vi "Write.vi"(8 "error in (no error)":errorcluster, 10 "Statement":T1={"timestamp"=timestamp(0 s since 1904-01-01), "level"=enum."INFO", "sourceTag"="", "originVI"="", "message"=""}, 11 "RelayAppender in":refnum<class "RelayAppender.lvclass">) -> (0 "error out":errorcluster, 3 "RelayAppender out":refnum<class "RelayAppender.lvclass">)   [LabVIEW 2026, in "Lumberjack.lvlib" / "RelayAppender.lvclass"]
doc: "Deliver one accepted Statement to the sink. Called by HandleStatement after the statement passes the appender threshold and filter. Receives the structured Statement (not a formatted string): text sinks format via their own Layout here; the relay forwards or enqueues the Statement object. Abstract. DD, must override."
uses:
  RelayAppender.lvclass
  TypeDefs/Statement.ctl
  TypeDefs/Severity.ctl
  RelayAppender.lvclass/RelayAppender.ctl
  Messages/LogStatementMsg.lvclass/LogStatementMsg.lvclass
  Lumberjack.lvlib
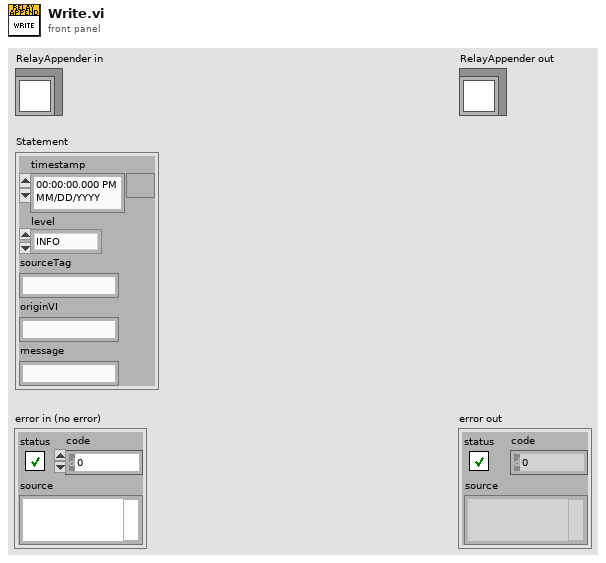
[diagram p1: front panel]
types:
  T1 = typedef "Lumberjack.lvlib/Statement.ctl" = cluster{"timestamp":timestamp, "level":T2, "sourceTag":string, "originVI":string, "message":string}
  T2 = typedef "Lumberjack.lvlib/Severity.ctl" = enum16{"OFF", "FATAL", "ERROR", "WARN", "INFO", "DEBUG", "TRACE", "ALL"}
  T3 = typedef "Lumberjack.lvlib/RelayMode.ctl" = enum16{"Message", "Queue"}
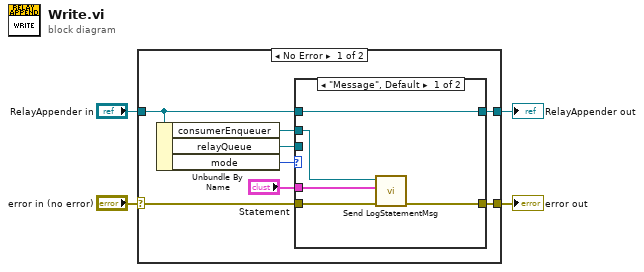
[diagram p0: block diagram]
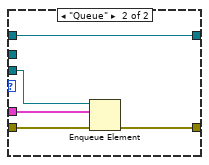
[diagram p2: hidden frame]
diagram:
  n1 = case shown="No Error" "error in (no error)" {
    selector: "error in (no error)" -> [w7 w24]
    tunnel: [w6 w24] -> w4
    tunnel: [w11 w23] -> w3
    tunnel: "RelayAppender in" -> [w12 w23]
    frame No Error {
      n2 = Unbundle By Name(w12) -> ("consumerEnqueuer"=w9:refnum<class "Message Enqueuer.lvclass">, "relayQueue"=w8:refnum<queue>, "mode"=w10:T3)
      n3 = case shown="\"Message\", Default" w10 {
        tunnel: w12 -> [w17 w22]
        tunnel: [w17 w22] -> w11
        tunnel: w9 -> [w15 _]
        tunnel: w8 -> [_ w18]
        tunnel: w7 -> [w16 w20]
        tunnel: [w13 w21] -> w6
        tunnel: "Statement" -> [w14 w19]
        frame "Message", Default {
          n4 = call "Send LogStatementMsg.vi"("error in (no error)"=w16, "Statement"=w14, "Enqueuer in"=w15) -> ("error out"=w13:errorcluster)  [unwired: 7 in, 1 out]
        }
        frame "Queue" {
          n5 = Enqueue Element(queue=w18, element=w19, error in (no error)=w20) -> (error out=w21:errorcluster)  [unwired: 1 in, 2 out]
        }
      }
    }
    frame Error {
    }
  }
  "error out" <- w4
  "RelayAppender out" <- w3
